vi "DS11202Z FrequencyCounting.vi"(10 "通道":enum16{"Channel_1", "Channel_2"}(ring), 11 "TestIndex":i32) -> (0 "错误输出":errorcluster, 3 "Value":dbl)   [LabVIEW 2015]
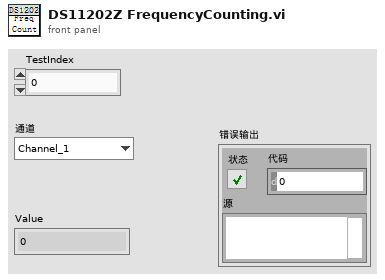
[diagram p1: front panel]
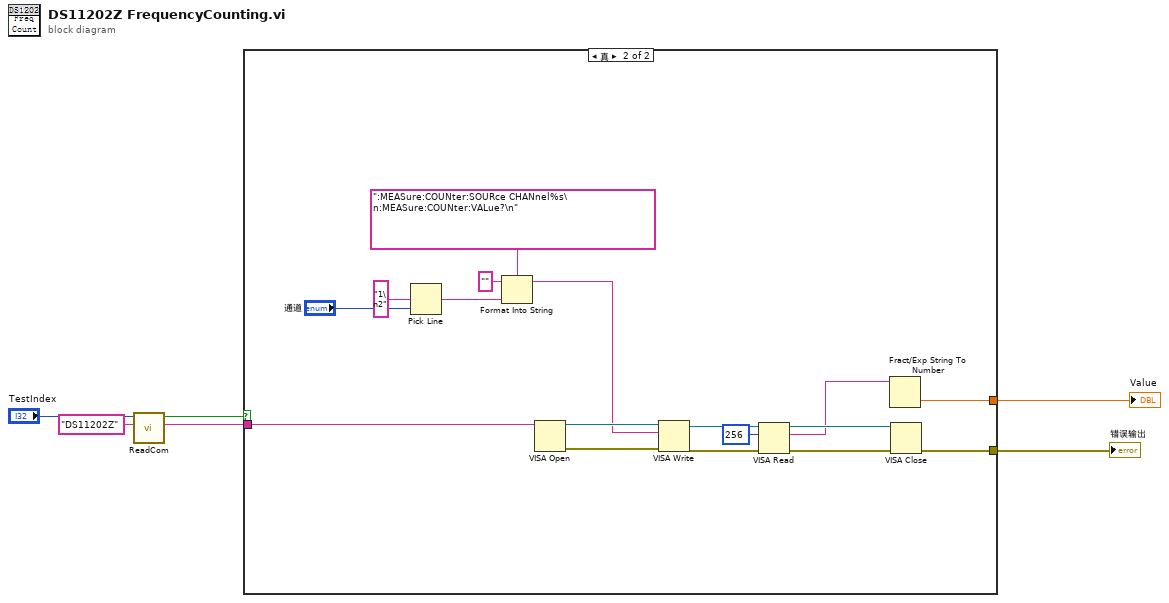
[diagram p0: block diagram]
diagram:
  n1 = call "ReadCom.vi"("仪器名称"="DS11202Z", "MyIndex"="TestIndex") -> ("COM"=w1:string, "OK?"=w2:bool)  [unwired: 7 in, 1 out]
  n2 = case shown="真" w2 {
    tunnel: [_ w18] -> w6
    tunnel: [_ w8] -> w5
    tunnel: w1 -> [_ w7]
    frame False {
    }
    frame True {
      n3 = Pick Line(multi-line string="1\n2", line index="通道") -> (output string=w21:string)  [unwired: 1 in]
      n4 = Format Into String(format string=":MEASure:COUNter:SOURce CHANnel%s\n:MEASure:COUNter:VALue?\n" ("字符串"), initial string="" ("初始字符串"), w21) -> (resulting string=w10:string)  [unwired: 1 in, 1 out]
      n5 = VISA Open(VISA resource name=w7) -> (VISA resource name=w20:refnum<visa-resource-name>, error out=w19:errorcluster)  [unwired: 1 in, 3 out]
      n6 = VISA Write(VISA resource name=w20, write buffer=w10, error in (no error)=w19) -> (VISA resource name out=w15:refnum<visa-resource-name>, error out=w17:errorcluster)  [unwired: 1 out]
      n7 = VISA Read(VISA resource name=w15, byte count=u32 256 ("字节总数"), error in (no error)=w17) -> (VISA resource name out=w14:refnum<visa-resource-name>, read buffer=w9:string, error out=w16:errorcluster)  [unwired: 1 out]
      n8 = Fract/Exp String To Number(string=w9) -> (number=w8:dbl)  [unwired: 3 in, 1 out]
      n9 = VISA Close(VISA resource name=w14, error in (no error)=w16) -> (error out=w18:errorcluster)
    }
  }
  "错误输出" <- w6
  "Value" <- w5
